vi "Gen Mixture Strings.vi"(9 "Mix Cluster":T1={"Ratio"=[0.6, 0.5], "Mix 2"=[12, 12], "Mix 1"=[0, 1]} {"Mix 1" items=["A1"=0, "A2"=1, "A3"=2, "A4"=3, "A5"=12]; "Mix 2" items=["B5"=8, "B6"=9, "B7"=10, "B8"=11, "A5"=12]}, 10 "Mix 2 Odors":string[](array[string]), 11 "Mix 1 Odors":string[](array[string])) -> (2 "mixture seq for logfile":string[][](array[string]), 3 "mixture sequence array":string[](array[string]))   [LabVIEW 2016]
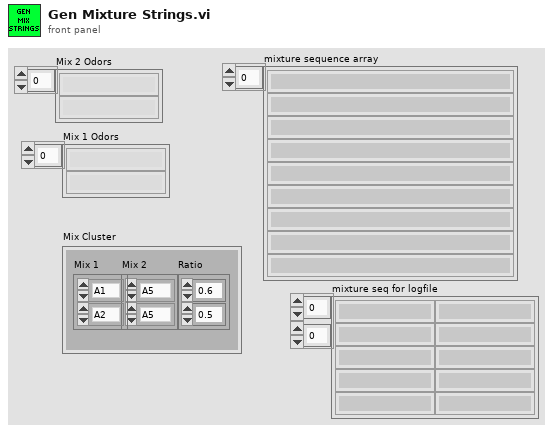
[diagram p1: front panel]
types:
  T1 = cluster{"Ratio":dbl[], "Mix 2":u16[], "Mix 1":u16[]}
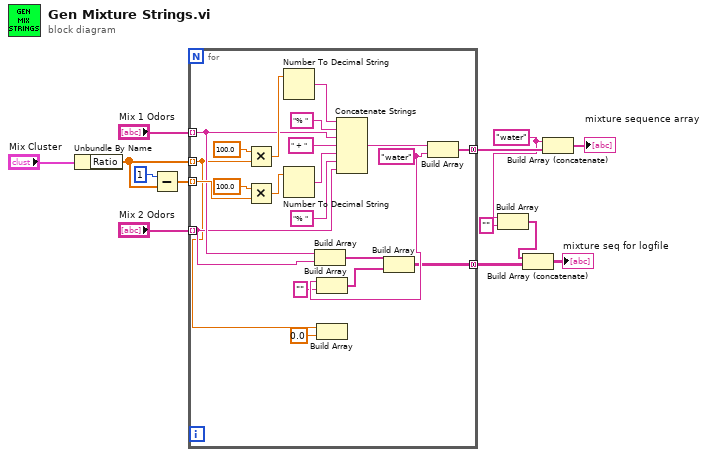
[diagram p0: block diagram]
diagram:
  w4 = "water" ("element")
  n1 = Unbundle By Name("Mix Cluster") -> ("Ratio"=w9:dbl[])
  n2 = Subtract(x=1, y=w9) -> (x-y=w8:dbl[])
  n3 = for {
    tunnel: "Mix 1 Odors" -> [w22] mode=indexing
    tunnel: "Mix 2 Odors" -> [w21] mode=indexing
    tunnel: w9 -> [w20] mode=indexing
    tunnel: w8 -> [w32] mode=indexing
    tunnel: [w23] -> w7 mode=concatenating
    tunnel: [w14] -> w5 mode=concatenating
    w17 = "water" ("element")
    n4 = Multiply(x=100.0, y=w20) -> (x*y=w31:dbl)
    n5 = Multiply(x=100.0, y=w32) -> (x*y=w30:dbl)
    n6 = Number To Decimal String(number=w31) -> (decimal integer string=w29:string)  [unwired: 1 in]
    n7 = Number To Decimal String(number=w30) -> (decimal integer string=w26:string)  [unwired: 1 in]
    n8 = Build Array(w22, w21) -> (w18:string[])
    n9 = Build Array(w17, "" ("element")) -> (w15:string[])
    n10 = Build Array(w20, 0.0 ("element")) -> ()  [unwired: 1 out]
    n11 = Concatenate Strings(w29, "% " ("string"), w22, " + " ("string"), w26, "% " ("string"), w21) -> (w24:string)
    n12 = Build Array(w18, w15) -> (w14:string[][])
    n13 = Build Array(w24, w17) -> (w23:string[])
  }
  n14 = Build Array(w4, "" ("element")) -> (w2:string[])
  n15 = Build Array (concatenate)(w2, w5) -> (→"mixture seq for logfile":string[][])
  n16 = Build Array (concatenate)(w4, w7) -> (→"mixture sequence array":string[])
